vi "small_RT Main.vi"() -> ()   [LabVIEW 2019]
doc: "Demonstrates the use of the Network Streams functions to receive LED status from the host computer."
uses:
  <vilib>/myRIO/Instrument Drivers/Onboard IO/DIO/typedefs/DIO Reference.ctl
  <vilib>/myRIO/Common/Instrument Driver Framework/Utilities/typedefs/myRIO Generic Hardware Reference.ctl
  <vilib>/myRIO/Common/Instrument Driver Framework/Utilities/typedefs/Hardware Version Enum.ctl
  <vilib>/myRIO/Common/Instrument Driver Framework/Utilities/typedefs/myRIO v1.0 Reference.ctl
  <vilib>/myRIO/Common/Instrument Driver Framework/Utilities/typedefs/Generic FPGA Reference.ctl
  <vilib>/myRIO/Common/Instrument Driver Framework/myRIO v1.0/DIO/typedefs/DIO Channels List.ctl
  <vilib>/myRIO/Common/Instrument Driver Framework/myRIO v1.0/DIO/typedefs/DIO Channels Enum.ctl
  <vilib>/userdefined/High Color/nirio_resource_hc.ctl
  <vilib>/myRIO/Common/Instrument Driver Framework/Utilities/vis/Is FPGA Ref Available.vi
  <vilib>/myRIO/Common/Instrument Driver Framework/myRIO v1.0/DIO/vis/myRIO v1.1 Open DIO.vi
  <vilib>/myRIO/Instrument Drivers/Onboard IO/DIO/vis/Write.vi
  <vilib>/myRIO/Common/Instrument Driver Framework/Utilities/vis/Validate Channels.vi
  <vilib>/myRIO/Common/Instrument Driver Framework/myRIO v1.0/DIO/vis/myRIO v1.0 Reserve DIO.vi
  <vilib>/myRIO/Common/Instrument Driver Framework/myRIO v1.0/UART/vis/myRIO v1.0 Close UART.vi
  <vilib>/myRIO/Common/Instrument Driver Framework/myRIO v1.0/Resource Manager/vis/myRIO v1.0 Reserve Channel List.vi
  <vilib>/myRIO/Common/Instrument Driver Framework/myRIO v1.0/DIO/vis/myRIO v1.0 Build MUX Configuration DIO.vi
  <vilib>/myRIO/Common/Instrument Driver Framework/myRIO v1.0/Resource Manager/vis/myRIO v1.0 Reserve Channel.vi
  <vilib>/myRIO/Common/Instrument Driver Framework/myRIO v1.0/Resource Manager/vis/myRIO v1.0 Unreserve Channel.vi
  <vilib>/myRIO/Common/Instrument Driver Framework/myRIO v1.0/Resource Manager/vis/myRIO v1.0 Create Configuration List.vi
  <vilib>/myRIO/Common/Instrument Driver Framework/myRIO v1.0/Resource Manager/vis/myRIO v1.0 Build Mutex Name.vi
  <vilib>/myRIO/Common/Instrument Driver Framework/Utilities/vis/FPGA Ref Manager.vi
  <vilib>/myRIO/Common/Instrument Driver Framework/myRIO v1.0/myRIO v1.0 Reset FPGA.vi
  <vilib>/myRIO/Common/Instrument Driver Framework/myRIO v1.0/IRQ/vis/myRIO v1.0 IRQ Info FGV.vi
  <vilib>/myRIO/Common/Instrument Driver Framework/myRIO v1.0/IRQ/vis/myRIO v1.0 Timer IRQ Info FGV.vi
  <vilib>/myRIO/Common/Instrument Driver Framework/myRIO v1.0/IRQ/vis/myRIO v1.0 ISR Agent.vi
  <vilib>/myRIO/Instrument Drivers/Utilities/vis/Reset Index.vi
  <vilib>/myRIO/Common/Instrument Driver Framework/myRIO v1.0/Resource Manager/vis/myRIO v1.0 Block Write Resource Manager.vi
  <vilib>/Utility/VariantDataType/GetNumericInfo.vi
  <vilib>/Utility/error.llb/Error Cluster From Error Code.vi
  <vilib>/myRIO/Common/Instrument Driver Framework/myRIO v1.0/myRIO v1.1 Open.vi
  <vilib>/myRIO/Common/Instrument Driver Framework/Utilities/vis/IO Manager.vi
  <vilib>/myRIO/Common/Instrument Driver Framework/Utilities/vis/Configuration Manager.vi
  <vilib>/myRIO/Common/Instrument Driver Framework/myRIO v1.0/Resource Manager/vis/myRIO v1.0 Configure IO.vi
  <vilib>/myRIO/Common/Instrument Driver Framework/myRIO v1.0/myRIO v1.0 Close.vi
  <vilib>/myRIO/Common/Instrument Driver Framework/myRIO v1.0/DIO/vis/myRIO v1.0 Write DIO.vi
  <vilib>/ErrorRing/Error Ring.xnode
  <vilib>/myRIO/Express VI/Onboard IO/DO/DO Express VI.xnode
  <vilib>/myRIO/Instrument Drivers/Onboard IO/DIO/vis/myRIO DIO Open.xnode
  <vilib>/myRIO/Instrument Drivers/Utilities/Utilities.lvlib
  <vilib>/myRIO/Instrument Drivers/Onboard IO/DIO/DIO.lvlib
panel:
  out "DIR":bool
  out "PUL":bool
  out "loops 2":i32
  out "delay time (ms)":dbl
  out "Stop_field":bool
  out "s":dbl format="%.3f"
  out "field error":errorcluster
  out "Receive":dbl[](array[numeric])
  out "loops":dbl
  out "error out":errorcluster
  in  "Stop":bool
  # "Overview: Demonstrates the use of the Network Streams functions to receive LED status from the host computer.\nInstructions:\n1. Run this VI.\n2. Open RT Main.vi and follow its front panel instructions.\n3. Click Stop to stop this VI. Stopping this VI also terminates the running of Desktop Main.vi."
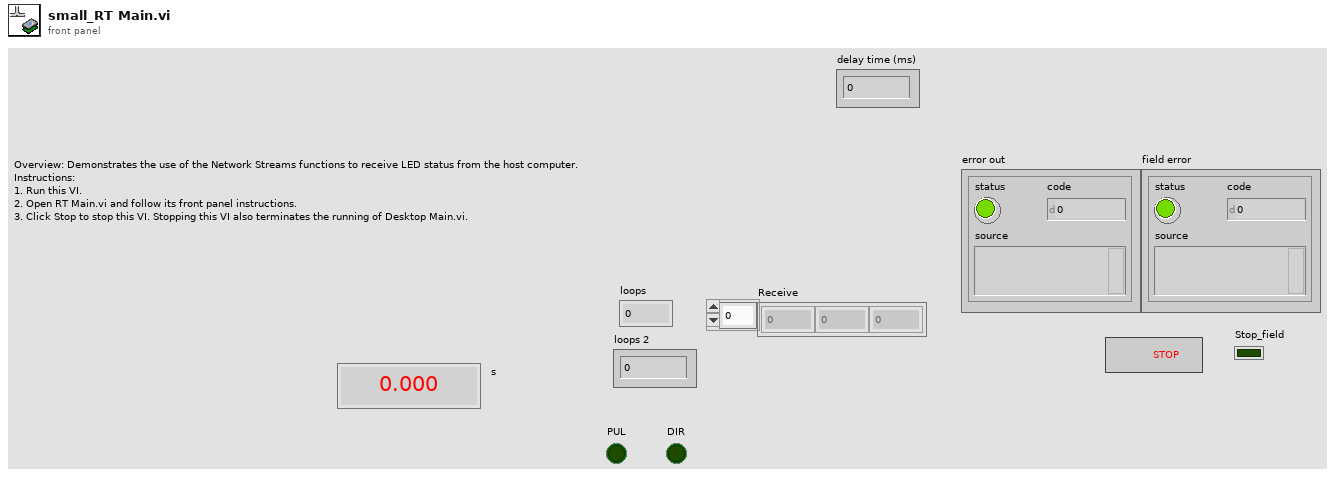
[diagram p1: front panel]
types:
  T1 = typedef "DIO.lvlib/DIO Reference.ctl" = cluster{"myRIO Reference":T2, "DIO Channels List":T6}
  T2 = typedef "myRIO Generic Hardware Reference.ctl" = cluster{"myRIO Model":T3, "myRIO Hardware Reference":T4}
  T3 = typedef "Hardware Version Enum.ctl" = enum16{"Unknown", "myRIO-1900", "myRIO-1950", "roboRIO", "NI ELVIS RIO CM", "ELVIS III"}
  T4 = typedef "myRIO v1.0 Reference.ctl" = cluster{"Generic FPGA Reference":T5, "Allow multiple opens":bool}
  T5 = typedef "Generic FPGA Reference.ctl" = refnum<k20>
  T6 = typedef "DIO Channels List.ctl" = T7[]
  T7 = typedef "DIO Channels Enum.ctl" = enum16{"Not Connected", "C/DIO0", "C/DIO1", "C/DIO2", "C/DIO3", "C/DIO4", "C/DIO5", "C/DIO6", "C/DIO7", "A/DIO0", "A/DIO1", "A/DIO2", "A/DIO3", "A/DIO4", "A/DIO5", "A/DIO6", "A/DIO7", "A/DIO8", "A/DIO9", "A/DIO10", "A/DIO11", "A/DIO12", "A/DIO13", "A/DIO14", "A/DIO15", "A/DIO16", "A/DIO17", "A/DIO18", "A/DIO19", "B/DIO0", "B/DIO1", "B/DIO2", "B/DIO3", "B/DIO4", "B/DIO5", "B/DIO6", "B/DIO7", "B/DIO8", "B/DIO9", "B/DIO10", "B/DIO11", "B/DIO12", "B/DIO13", "B/DIO14", "B/DIO15", "B/DIO16", "B/DIO17", "B/DIO18", "B/DIO19", "LED0", "LED1", "LED2", "LED3", "Button0", "DIO/DIO0", "DIO/DIO1", "DIO/DIO2", "DIO/DIO3", "DIO/DIO4", "DIO/DIO5", "DIO/DIO6", "DIO/DIO7", "DIO/DIO8", "DIO/DIO9", "SPI/CS0", "SPI/CS1", "SPI/CS2", "SPI/CS3", "LED RADIO (Green)", "LED RADIO (Red)", "LED COMM (Green)", "LED COMM (Red)", "LED MODE (Green)", "LED MODE (Red)"}
  T8 = typedef "nirio_resource_hc.ctl" = tag
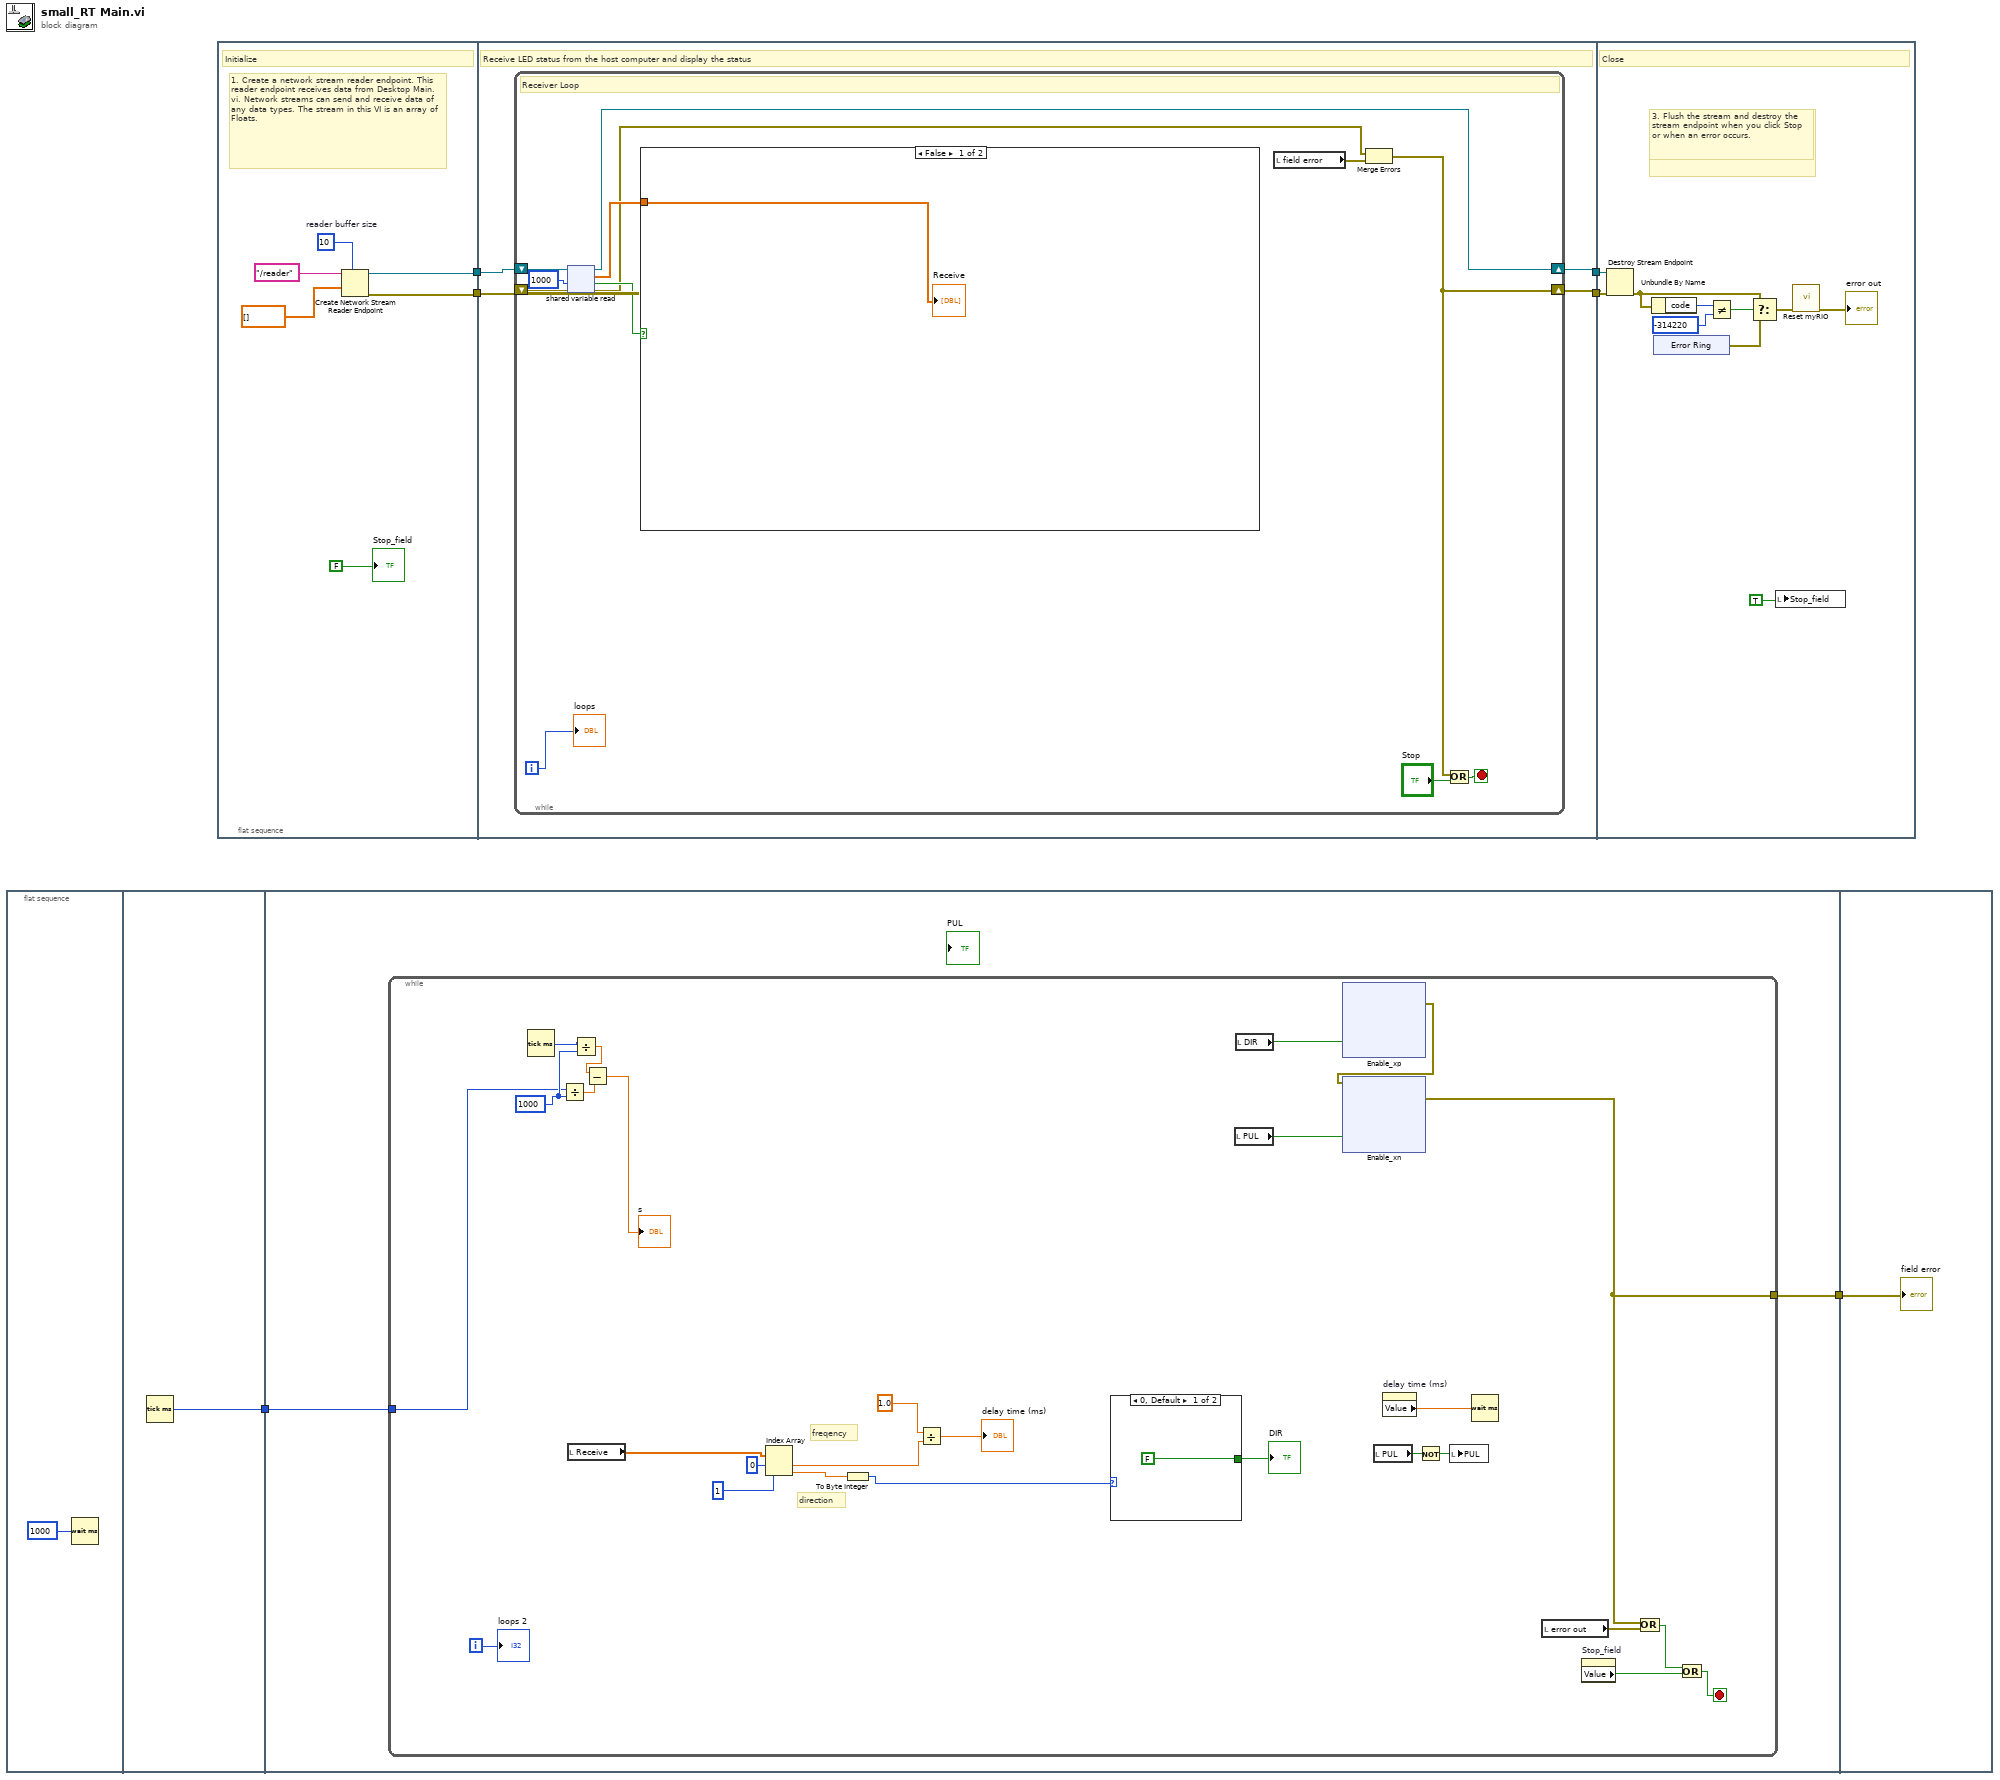
[diagram p0: block diagram]
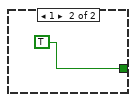
[diagram p2: hidden frame]
diagram:
  n1 = flat-sequence {
    tunnel: [w8] -> w2
    tunnel: w2 -> [w10]
    tunnel: [w9] -> w1
    tunnel: w1 -> [w110]
    frame #0 {
      n2 = Wait (ms)(milliseconds to wait=1000) -> ()  [unwired: 1 out]
    }
    frame #1 {
      n3 = Tick Count (ms)() -> (millisecond timer value=w8:u32)
    }
    frame #2 {
      n4 = while {
        tunnel: w10 -> [w31]
        tunnel: [w26] -> w9
        i -> [w25]
        stop <- w37 stop-if-true
        w34 = 1000
        # "direction"
        # "freqency"
        n5 = Tick Count (ms)() -> (millisecond timer value=w35:u32)
        n6 = Divide(x=w31, y=w34) -> (x/y=w36:dbl)
        n7 = local read "Receive"() -> (w23:dbl[])
        n8 = Divide(x=w35, y=w34) -> (x/y=w33:dbl)
        n9 = Subtract(x=w33, y=w36) -> (x-y=→"s":dbl)
        n10 = Index Array(array=w23, index #1=0 ("index"), index #2=1 ("index")) -> (element #1=w21:dbl, element #2=w20:dbl)
        n11 = To Byte Integer(number=w20) -> (8bit integer=w24:i8)
        n12 = Divide(x=1.0, y=w21) -> (x/y=→"delay time (ms)":dbl)
        n13 = case shown="0, Default" w24 {
          tunnel: [FALSE TRUE ("DIR")] -> w11
          frame 0, Default {
          }
          frame 1 {
          }
        }
        "DIR" <- w11
        n14 = local read "PUL"() -> (w12:bool)
        n15 = local read "DIR"() -> (w13:bool)
        n16 = xnode "Enable_xp"("B/DIO0 (Pin 11)"=w13) -> ("error out"=w32:errorcluster)  [unwired: 1 in]
        n17 = xnode "Enable_xn"("B/DIO1 (Pin 13)"=w12, "error in (no error)"=w32) -> ("error out"=w26:errorcluster)
        n18 = local read "PUL"() -> (w16:bool)
        n19 = property on="delay time (ms)" class="DigNum (strict)"() -> ("Value"=w14:dbl)  [unwired: 2 in, 2 out]
        n20 = Not(x=w16) -> (.not. x?=w15:bool)
        n21 = local write "PUL"(w15) -> ()
        n22 = Wait (ms)(milliseconds to wait=w14) -> ()  [unwired: 1 out]
        n23 = local read "error out"() -> (w30:errorcluster)
        n24 = property on="Stop_field" class="Bool (strict)"() -> ("Value"=w28:bool)  [unwired: 2 in, 2 out]
        n25 = Or(x=w26, y=w30) -> (x .or. y?=w29:bool)
        n26 = Or(x=w29, y=w28) -> (x .or. y?=w37:bool)
        "loops 2" <- w25
      }
    }
    frame #3 {
      "field error" <- w110
    }
  }
  n27 = flat-sequence {
    tunnel: [w114] -> w3
    tunnel: [w113] -> w4
    tunnel: [w117] -> w6
    tunnel: [w118] -> w5
    tunnel: w3 -> [w120]
    tunnel: w4 -> [w119]
    tunnel: w6 -> [w143]
    tunnel: w5 -> [w142]
    frame #0 {
      w116 = 10  # reader buffer size
      # "1. Create a network stream reader endpoint. This reader endpoint receives data from Desktop Main.vi. Network streams can send and receive data of any data types. The stream in this VI is an array of Floats."
      # "Initialize"
      n28 = Create Network Stream Reader Endpoint(7:w116, 9:dbl[] [], 11:"/reader" ("reader name")) -> (0:w113:errorcluster, 3:w114:refnum<k21>)  [unwired: 4 in]
      "Stop_field" <- FALSE
    }
    frame #1 {
      # "Receive LED status from the host computer and display the status"
      n29 = while {
        shift-right: [w127] -> w117
        shift-left: w120 -> [w128]
        shift-right: [w122] -> w118
        shift-left: w119 -> [w130]
        i -> [w126]
        stop <- w131 stop-if-true
        # "Receiver Loop"
        n30 = shared-variable-read(w128, w130, 1000 ("timeout ms (-1)")) -> (w127:refnum<k21>, w121:errorcluster, w125:bool, w124:dbl[])
        n31 = case shown="False" w125 {
          tunnel: w124 -> [w133 _]
          frame False {
            "Receive" <- w133
          }
          frame True {
            # "time out occurs, no data is received"
          }
        }
        n32 = local read "field error"() -> (w123:errorcluster)
        n33 = Merge Errors(w121, w123) -> (w122:errorcluster)
        n34 = Or(x=w122, y="Stop") -> (x .or. y?=w131:bool)
        "loops" <- w126
      }
    }
    frame #2 {
      # "4. Error -314220 indicates that the other endpoint has been destroyed. This VI ignores this error."
      # "3. Flush the stream and destroy the stream endpoint when you click Stop or when an error occurs."
      # "Close"
      n35 = Destroy Stream Endpoint(8:w142, 11:w143) -> (0:w137:errorcluster)
      n36 = Unbundle By Name(w137) -> ("code"=w141:i32)
      n37 = xnode "Error Ring"() -> ("error out"=w138:errorcluster)
      n38 = Not Equal?(x=w141, y=-314220) -> (x != y?=w139:bool)
      n39 = Select(t=w137, s=w139, f=w138) -> (s? t:f=w136:errorcluster)
      n40 = local write "Stop_field"(TRUE) -> ()
      n41 = call <vilib>:"Reset myRIO.vi"("error in (no error)"=w136) -> ("error out"=→"error out":errorcluster)  [unwired: 10 in]
    }
  }
